vi "矩形缩放（TB）.vi"(10 "缩放偏移量":cluster{"x":i16, "y":i16} caption="点", 11 "矩形":T1) -> (3 "缩放后矩形":T1)   [LabVIEW 2011]
uses:
  RectTB.ctl
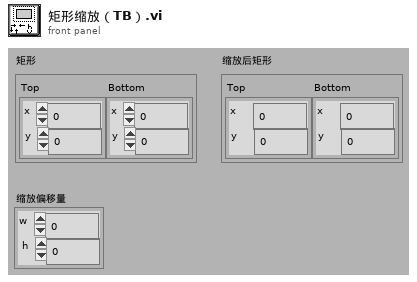
[diagram p1: front panel]
types:
  T1 = typedef "RectTB.ctl" = cluster{"Top":cluster{"x":i16, "y":i16}, "Bottom":cluster{"x":i16, "y":i16}}
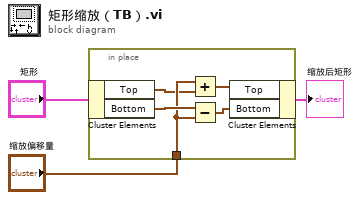
[diagram p0: block diagram]
diagram:
  n1 = in-place {
    in-place-border: "缩放偏移量" -> [w6]
    n2 = in-place-cluster #1("矩形") -> ("Top"=w5:cluster{"x":i16, "y":i16}, "Bottom"=w8:cluster{"x":i16, "y":i16})
    n3 = Add(x=w6, y=w5) -> (x+y=w4:cluster{"x":i16, "y":i16})
    n4 = Subtract(x=w8, y=w6) -> (x-y=w7:cluster{"x":i16, "y":i16})
    n5 = in-place-cluster #1("Top"=w4, "Bottom"=w7) -> (→"缩放后矩形":T1)
  }
